vi "from string array.vi"(8 "error in (no error)":errorcluster, 9 "String Array":string[][](array[string]), 10 "version":string, 11 "Benchmark PID configuration in":refnum<class "Benchmark PID configuration.lvclass">) -> (0 "error out":errorcluster, 3 "Benchmark PID configuration out":refnum<class "Benchmark PID configuration.lvclass">)   [LabVIEW 2018, in "Benchmark PID configuration.lvclass"]
uses:
  Benchmark PID configuration.lvclass
  Line.ctl
  <vilib>/NI/Tag Bus Module Framework/channel/TBM channel.lvclass
  Benchmark PID configuration.lvclass/Benchmark PID configuration.ctl
  Write Lines.vi
  Get Line Name.vi
  <vilib>/NI/Tag Bus Module Framework/module configuration/FindDuplicate.vi
  <vilib>/Utility/error.llb/Error Cluster From Error Code.vi
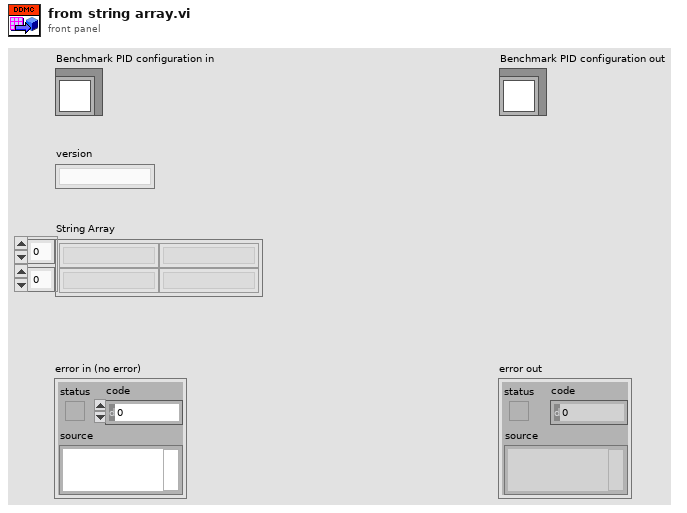
[diagram p1: front panel]
types:
  T1 = typedef "Benchmark PID configuration.lvclass/Line.ctl" = cluster{"PID Name":string, "Setpoint":refnum<class "TBM channel.lvclass">, "Variable":refnum<class "TBM channel.lvclass">, "Output":refnum<class "TBM channel.lvclass">}
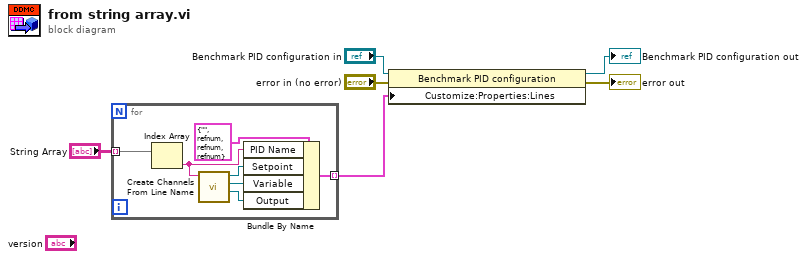
[diagram p0: block diagram]
diagram:
  n1 = for {
    tunnel: "String Array" -> [w13] mode=indexing
    tunnel: [w12] -> w1 mode=indexing
    n2 = Index Array(array=w13) -> (element=w10:string)  [unwired: 1 in]
    n3 = call "Create Channels From Line Name.vi"("String"=w10) -> ("channel"=w7:refnum<class "TBM channel.lvclass">, "channel 2"=w8:refnum<class "TBM channel.lvclass">, "TBM channel out"=w9:refnum<class "TBM channel.lvclass">)  [unwired: 8 in]
    n4 = Bundle By Name(cluster=T1 {"PID Name"="", "Setpoint"=refnum, "Variable"=refnum, "Output"=refnum} ("Line"), "PID Name"=w10, "Setpoint"=w9, "Variable"=w8, "Output"=w7) -> (w12:T1)
  }
  n5 = property class="Benchmark PID configuration"(reference="Benchmark PID configuration in", error in="error in (no error)", "Customize:Properties:Lines"=w1) -> (reference out=→"Benchmark PID configuration out":refnum<class "Benchmark PID configuration.lvclass">, error out=→"error out":errorcluster)
